vi "convertGpsDifToDistance.vi"(9 "Location 2":cluster{"Latitude":dbl, "Longitude":dbl} {"Longitude" format="%.8g"; "Latitude" format="%.8g"}, 11 "Location 1":cluster{"Latitude":dbl, "Longitude":dbl} {"Longitude" format="%.8g"; "Latitude" format="%.8g"}) -> (1 "destance2 [m]":dbl format="%.3g", 3 "distance [m]":dbl format="%.3g")   [LabVIEW 2023]
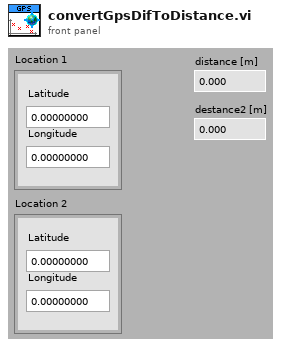
[diagram p1: front panel]
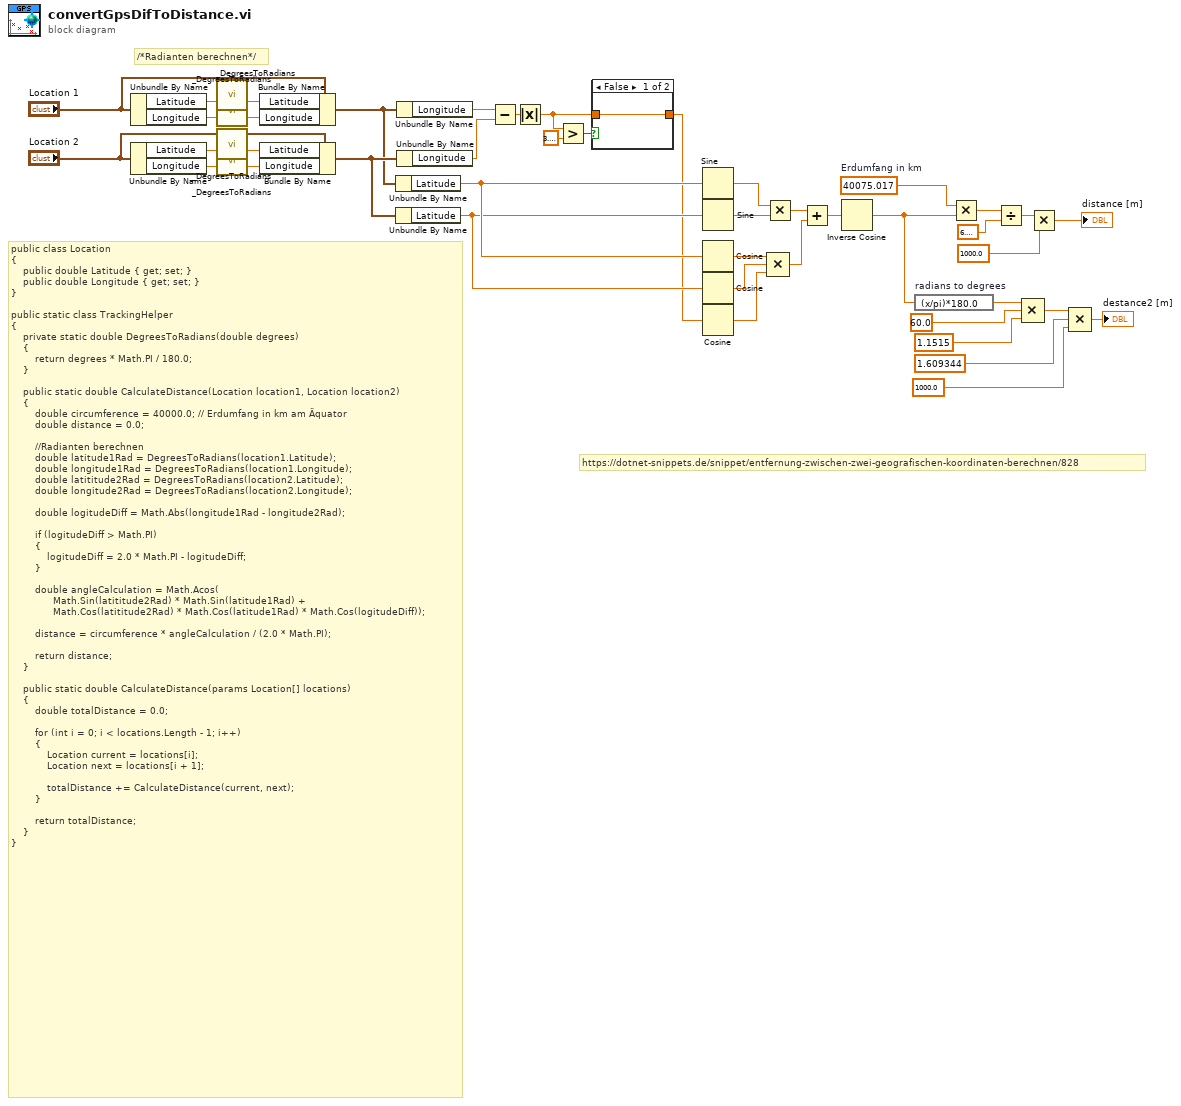
[diagram p0: block diagram]
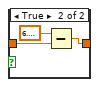
[diagram p2: hidden frame]
diagram:
  w19 = 40075.017  # Erdumfang in km
  # "https://dotnet-snippets.de/snippet/entfernung-zwischen-zwei-geografischen-koordinaten-berechnen/828"
  # "/*Radianten berechnen*/"
  # "public class Location\n{\n    public double Latitude { get; set; }\n    public double Longitude { get; set; }\n}\n\npublic static class TrackingHelper\n{\n    private static double DegreesToRadians(double degrees)\n    {\n        return degrees * Math.PI / 180.0;\n    }\n\n    public static double CalculateDistance(Location location1, Location location2)\n    {\n        double circumference = 40000.0; // Erdumfang in km am Äquator\n        double distance = 0.0;\n        \n        //Radianten berechnen\n        double latitude1Rad = DegreesToRadians(location1.Latitude);\n        double longitude1Rad = DegreesToRadians(location1.Longitude);\n        double latititude2Rad = DegreesToRadians(location2.Latitude);\n        double longitude2Rad = DegreesToRadians(location2.Longitude);\n\n        double logitudeDiff = Math.Abs(longitude1Rad - longitude2Rad);\n\n        if (logitudeDiff > Math.PI)\n        {\n            logitudeDiff = 2.0 * Math.PI - logitudeDiff;\n        }\n        \n        double angleCalculation = Math.Acos(\n              Math.Sin(latititude2Rad) * Math.Sin(latitude1Rad) +\n              Math.Cos(latititude2Rad) * Math.Cos(latitude1Rad) * Math.Cos(logitudeDiff));\n\n        distance = circumference * angleCalculation / (2.0 * Math.PI);\n\n        return distance;\n    }\n\n    public static double CalculateDistance(params Location[] locations)\n    {\n        double totalDistance = 0.0;\n\n        for (int i = 0; i < locations.Length - 1; i++)\n        {\n            Location current = locations[i];\n            Location next = locations[i + 1];\n\n            totalDistance += CalculateDistance(current, next);\n        }\n\n        return totalDistance;\n    }\n}"
  n1 = Unbundle By Name("Location 1") -> ("Latitude"=w4:dbl, "Longitude"=w3:dbl)
  n2 = Unbundle By Name("Location 2") -> ("Latitude"=w8:dbl, "Longitude"=w7:dbl)
  n3 = call "_DegreesToRadians.vi"("Degrees In"=w4) -> ("Radians"=w1:dbl)  [unwired: 14 in]
  n4 = call "_DegreesToRadians.vi"("Degrees In"=w3) -> ("Radians"=w2:dbl)  [unwired: 14 in]
  n5 = call "_DegreesToRadians.vi"("Degrees In"=w8) -> ("Radians"=w5:dbl)  [unwired: 14 in]
  n6 = call "_DegreesToRadians.vi"("Degrees In"=w7) -> ("Radians"=w6:dbl)  [unwired: 14 in]
  n7 = Bundle By Name(cluster="Location 1", "Latitude"=w1, "Longitude"=w2) -> (w34:cluster{"Latitude":dbl, "Longitude":dbl})
  n8 = Bundle By Name(cluster="Location 2", "Latitude"=w5, "Longitude"=w6) -> (w35:cluster{"Latitude":dbl, "Longitude":dbl})
  n9 = Unbundle By Name(w34) -> ("Latitude"=w31:dbl)
  n10 = Unbundle By Name(w35) -> ("Latitude"=w30:dbl)
  n11 = Unbundle By Name(w34) -> ("Longitude"=w41:dbl)
  n12 = Unbundle By Name(w35) -> ("Longitude"=w40:dbl)
  n13 = Subtract(x=w41, y=w40) -> (x-y=w39:dbl)
  n14 = Absolute Value(x=w39) -> (abs(x)=w36:dbl)
  n15 = Greater?(x=w36, y=3.141592653589793) -> (0:w37:bool)
  n16 = case shown="False" w37 {
    tunnel: w36 -> [w44 w47]
    tunnel: [w44 w45] -> w29
    frame False {
    }
    frame True {
      n17 = Subtract(x=6.283185307179586, y=w47) -> (x-y=w45:dbl)
    }
  }
  n18 = Sine(x=w31) -> (sin(x)=w33:dbl)
  n19 = Sine(x=w30) -> (sin(x)=w32:dbl)
  n20 = Cosine(x=w31) -> (cos(x)=w28:dbl)
  n21 = Cosine(x=w30) -> (cos(x)=w27:dbl)
  n22 = Cosine(x=w29) -> (cos(x)=w26:dbl)
  n23 = Multiply(x=w33, y=w32) -> (x*y=w25:dbl)
  n24 = Compound Arithmetic op=MULTIPLY(w28, w27, w26) -> (w24:dbl)
  n25 = Add(x=w25, y=w24) -> (x+y=w23:dbl)
  n26 = Inverse Cosine(1:w23) -> (0:w11:dbl)
  n27 = expression code="(x/pi)*180.0" "radians to degrees"(w11) -> (w18:dbl)
  n28 = Multiply(x=w19, y=w11) -> (x*y=w22:dbl)
  n29 = Divide(x=w22, y=6.283185307179586) -> (x/y=w20:dbl)
  n30 = Compound Arithmetic op=MULTIPLY(w18, 60.0 ("value"), 1.1515 ("value")) -> (w15:dbl)
  n31 = Multiply(x=w20, y=1000.0 ("x")) -> (x*y=→"distance [m]":dbl)
  n32 = Compound Arithmetic op=MULTIPLY(w15, 1.609344 ("value"), 1000.0 ("value")) -> (→"destance2 [m]":dbl)
